vi "Normalize Decay.vi"(9 "IRF (F)":bool, 11 "Decay":cluster{"t Array":dbl[], "Y Array":dbl[]}) -> (0 "Step":dbl, 1 "Normalization Factor":dbl, 3 "Normalized Decay":cluster{"t Array":dbl[], "Y Array":dbl[]})   [LabVIEW 2021, in "Fits.lvlib"]
doc: "Normalizes the incoming plot such that the integral equals 1.\n\n* <B>IRF = False</B>: The Y Array is divided by the sum of all Y values (<B>Normalization Factor</B>) multiplied by the most likely abscissa step (<B>Step</B>, maximum interval between successive abscissa).\n\n* <B>IRF = True</B>: The Y Array is divided by the sum of all Y values (<B>Normalization Factor</B>)."
uses:
  Fits.lvlib
  c65b08c5-93fc-4e90-ad2d-ad135c1fbea9.vi
  63561826-c737-4851-a63c-e09521817127.vi
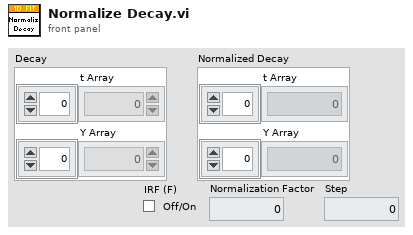
[diagram p1: front panel]
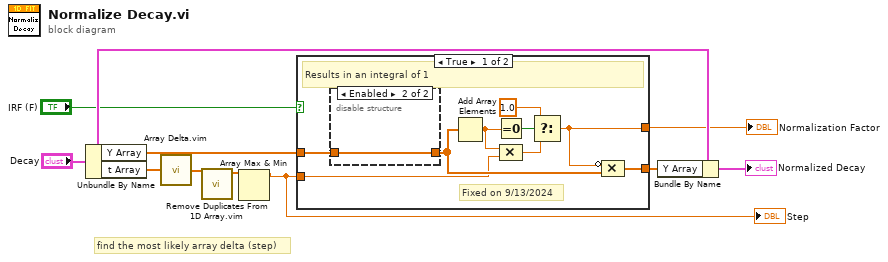
[diagram p0: block diagram]
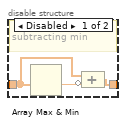
[diagram p2: hidden frame]
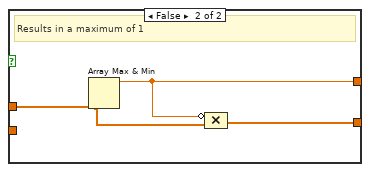
[diagram p3: hidden frame]
diagram:
  # "find the most likely array delta (step)"
  n1 = Unbundle By Name("Decay") -> ("Y Array"=w6:dbl[], "t Array"=w8:dbl[])
  n2 = call "Array Delta.vim"("A[i]"=w8) -> ("A[i+1]-A[i]"=w2:dbl[])  [unwired: 8 in]
  n3 = call "Remove Duplicates From 1D Array.vim"("array"=w2) -> ("array with duplicates removed"=w3:dbl[])  [unwired: 10 in]
  n4 = Array Max & Min(array=w3) -> (max value=w1:dbl)  [unwired: 3 out]
  "Step" <- w1
  n5 = case shown="True" "IRF (F)" {
    tunnel: [w19 w26] -> w7
    tunnel: w6 -> [w18 w25]
    tunnel: [w17 w24] -> w5
    tunnel: w1 -> [w11 _]
    frame True {
      # "Fixed on 9/13/2024"
      # "Results in an integral of 1"
      n6 = disable-structure shown="Enabled" {
        disable-tunnel: w18 -> [w21 w23]
        disable-tunnel: [w20 w23] -> w16
        frame Disabled {
          # "subtracting min"
          n7 = Array Max & Min(array=w21) -> (min value=w22:dbl)  [unwired: 3 out]
          n8 = Compound Arithmetic op=ADD(w21, invert w22) -> (w20:dbl[])
        }
        frame Enabled {
        }
      }
      n9 = Add Array Elements(numeric array=w16) -> (sum=w14:dbl)
      n10 = Equal To 0?(x=w14) -> (x = 0?=w15:bool)
      n11 = Compound Arithmetic op=MULTIPLY(w14, w11) -> (w12:dbl)
      n12 = Select(t=1.0, s=w15, f=w12) -> (s? t:f=w17:dbl)
      n13 = Compound Arithmetic op=MULTIPLY(invert w17, w16) -> (w19:dbl[])
    }
    frame False {
      # "find the most likely array delta (step)"
      # "Results in a maximum of 1"
      n14 = Array Max & Min(array=w25) -> (max value=w24:dbl)  [unwired: 3 out]
      n15 = Compound Arithmetic op=MULTIPLY(invert w24, w25) -> (w26:dbl[])
    }
  }
  "Normalization Factor" <- w5
  n16 = Bundle By Name(cluster="Decay", "Y Array"=w7) -> (→"Normalized Decay":cluster{"t Array":dbl[], "Y Array":dbl[]})
